vi "Configure Measurement.vi"(8 "error in (no error)":errorcluster, 10 "Measurement Settings":T1={"Function"=enum."DC Volts", "Resolution in Digits"=5.5, "Range"=0.02} {"Range" format="%.2f"; "Resolution in Digits" items=["3 1/2"=3.5, "4 1/2"=4.5, "5 1/2"=5.5, "6 1/2"=6.5, "7 1/2"=7.5]}, 11 "Session Handle":refnum<k15>) -> (0 "error out":errorcluster, 3 "Session Handle Out":refnum<k15>)   [LabVIEW 2026, in "PXI4072.lvlib"]
uses:
  PXI4072.lvlib
  Types/PXI4072 Settings.ctl
  <instrlib>/niDMM/nidmm.llb/niDMM Function.ctl
  <instrlib>/niDMM/nidmm.llb/niDMM Resolution in Digits.ctl
  <instrlib>/niDMM/nidmm.llb/niDMM Configure Measurement Digits.vi
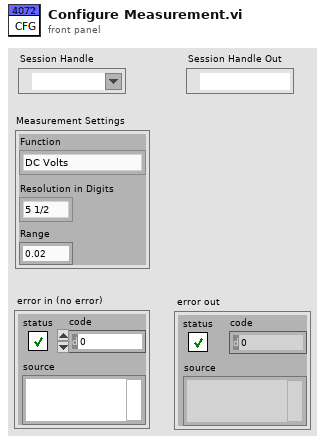
[diagram p1: front panel]
types:
  T1 = typedef "PXI4072.lvlib/PXI4072 Settings.ctl" = cluster{"Function":T2, "Resolution in Digits":T3, "Range":dbl}
  T2 = typedef "niDMM Function.ctl" = enum16{"DC Volts", "AC Volts", "DC Current", "AC Current", "2-wire Resistance", "4-wire Resistance", "Diode", "Frequency", "Period", "AC Volts DC Coupled", "Capacitance", "Inductance", "Temperature"}
  T3 = typedef "niDMM Resolution in Digits.ctl" = dbl
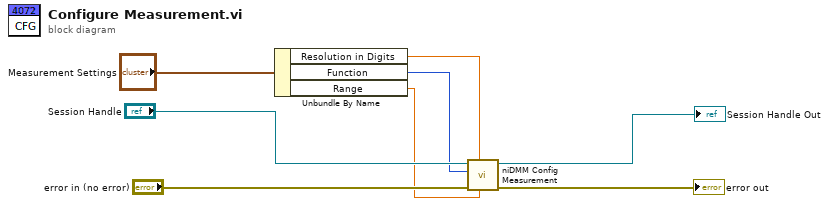
[diagram p0: block diagram]
diagram:
  n1 = Unbundle By Name("Measurement Settings") -> ("Resolution in Digits"=w3:T3, "Function"=w2:T2, "Range"=w1:dbl)
  n2 = call-poly <instrlib>:"niDMM Config Measurement.vi"("Range"=w1, "Resolution in Digits"=w3, "error in (no error)"="error in (no error)", "Function"=w2, "instrument handle"="Session Handle") -> ("error out"=→"error out":errorcluster, "instrument handle out"=→"Session Handle Out":refnum<k15>)  [unwired: 5 in]
